vi "Keithley 622x Program Voltmeter.vi"() -> ()   [LabVIEW 2021]
panel:
  out "read buffer":string
  in  "write buffer 2":string
  in  "write buffer":string
  in  "VISA resource name":refnum<visa-resource-name>
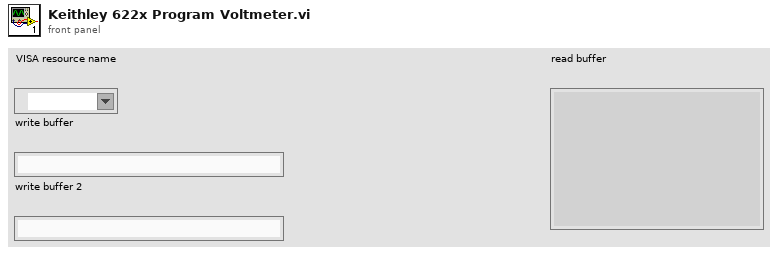
[diagram p1: front panel]
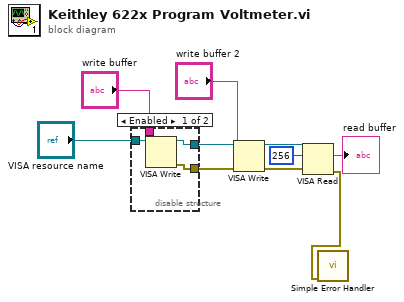
[diagram p0: block diagram]
diagram:
  n1 = disable-structure shown="Enabled" {
    disable-tunnel: "VISA resource name" -> [w14 w15]
    disable-tunnel: [w13 w15] -> w9
    disable-tunnel: "write buffer" -> [w12 _]
    disable-tunnel: [w11 _] -> w3
    frame Enabled {
      n2 = VISA Write(VISA resource name=w14, write buffer=w12) -> (VISA resource name out=w13:refnum<visa-resource-name>, error out=w11:errorcluster)  [unwired: 1 in, 1 out]
    }
    frame Disabled {
    }
  }
  n3 = VISA Write(VISA resource name=w9, write buffer="write buffer 2", error in (no error)=w3) -> (VISA resource name out=w8:refnum<visa-resource-name>, error out=w2:errorcluster)  [unwired: 1 out]
  n4 = VISA Read(VISA resource name=w8, byte count=u32 256, error in (no error)=w2) -> (read buffer=→"read buffer":string, error out=w1:errorcluster)  [unwired: 2 out]
  n5 = call <vilib>:"Simple Error Handler.vi"("error in (no error)"=w1) -> ()  [unwired: 4 in, 5 out]
